vi "LWXPS_EventWait.vi"(0 "XPS Reference IN":refnum<k24>, 5 "Positioner Name":string, 7 "Event Name":string, 9 "Event Parameter":string, 11 "LabVIEW error IN":errorcluster) -> (4 "XPS Reference OUT":refnum<k24>, 6 "Returned error code":i32, 8 "XPS Error String":string, 15 "LabVIEW error OUT":errorcluster)   [LabVIEW 2014]
uses:
  D:/XPSQ8_LabView_Library/Development/Source/Dll/Newport.XPS.CommandInterface.dll
  Dll/Newport.XPS.CommandInterface.dll
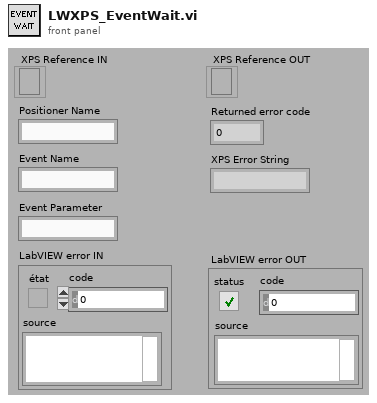
[diagram p1: front panel]
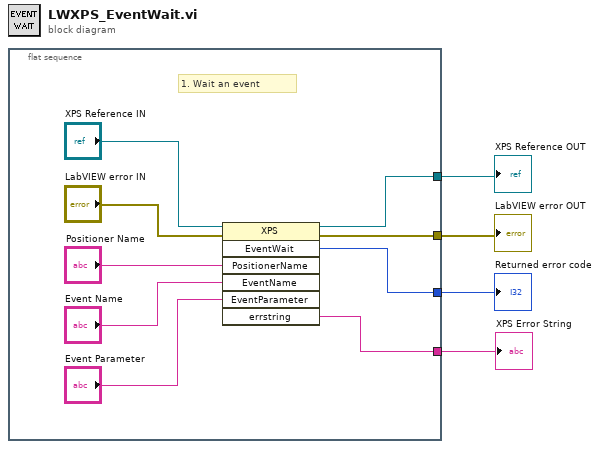
[diagram p0: block diagram]
diagram:
  n1 = flat-sequence {
    tunnel: [w11] -> w4
    tunnel: [w9] -> w3
    tunnel: [w10] -> w1
    tunnel: [w8] -> w2
    frame #0 {
      # "1. Wait an event"
      n2 = invoke class="XPS" method="EventWait"(reference="XPS Reference IN", error in="LabVIEW error IN", "PositionerName"="Positioner Name", "EventName"="Event Name", "EventParameter"="Event Parameter") -> (reference out=w11:refnum<k24>, error out=w9:errorcluster, "EventWait"=w10:i32, "errstring"=w8:string)  [unwired: 2 in, 3 out]
    }
  }
  "XPS Reference OUT" <- w4
  "LabVIEW error OUT" <- w3
  "XPS Error String" <- w2
  "Returned error code" <- w1
